vi "A TO V CONVERTER.vi"(8 "error in (no error)":errorcluster, 9 "A max Banco 2":dbl, 10 "A max Banco 1":dbl, 11 "Set Point":dbl) -> (0 "error out":errorcluster, 3 "Set Value to cDAQ":dbl)   [LabVIEW 2019]
uses:
  BenchSelector.vi
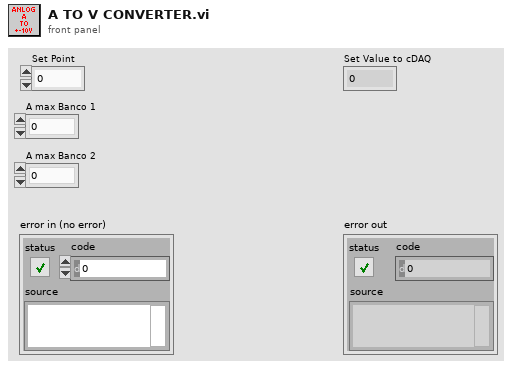
[diagram p1: front panel]
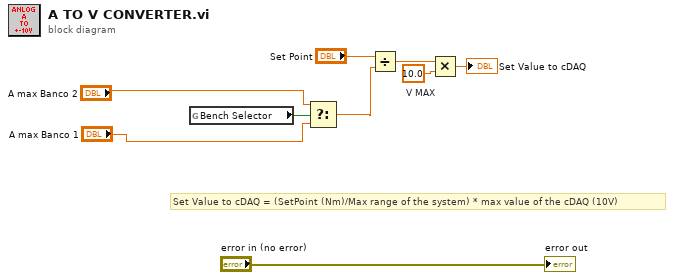
[diagram p0: block diagram]
diagram:
  w7 = 10.0  # V MAX
  # "Set Value to cDAQ = (SetPoint (Nm)/Max range of the system) * max value of the cDAQ (10V)"
  n1 = global read "BenchSelector.vi" "Bench Selector"() -> (w4:bool)
  n2 = Select(t="A max Banco 2", s=w4, f="A max Banco 1") -> (s? t:f=w3:dbl)
  n3 = Divide(x="Set Point", y=w3) -> (x/y=w8:dbl)
  n4 = Multiply(x=w8, y=w7) -> (x*y=→"Set Value to cDAQ":dbl)
  "error out" <- "error in (no error)"
